vi "initialize hmac.vi"(8 "error in":errorcluster, 10 "key":string, 11 "digest name":string) -> (0 "error out":errorcluster, 3 "lvlibcrypto digest out":refnum<class "lvlibcrypto digestsign.lvclass">)   [LabVIEW 2016, in "lvlibcrypto digestsign.lvclass"]
uses:
  lvlibcrypto digestsign.lvclass
  lv tls dll.lvlib
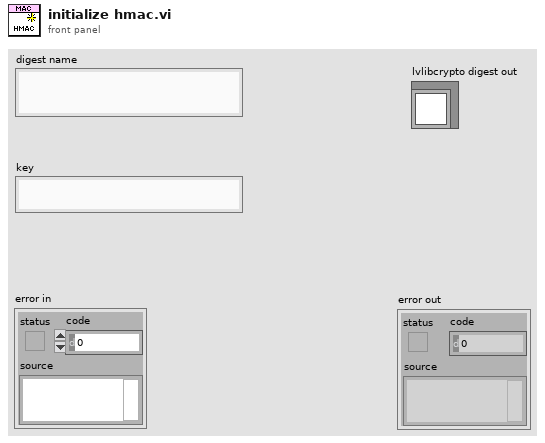
[diagram p1: front panel]
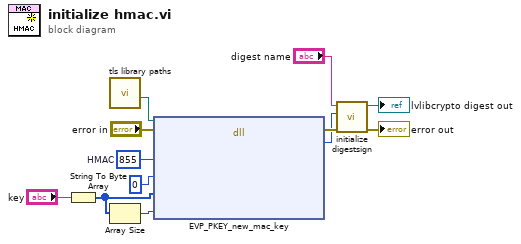
[diagram p0: block diagram]
diagram:
  w1 = 855  # HMAC
  n1 = String To Byte Array(string="key") -> (unsigned byte array=w3:u8[])
  n2 = call "tls library paths.vi"() -> ("libcrypto"=w9:path)  [unwired: 8 in, 3 out]
  n3 = Array Size(array=w3) -> (size(s)=w4:i32)
  n4 = dll-call lib="C:/Users/IEUser/Desktop/tlssimple/libcrypto-41.dll" fn="EVP_PKEY_new_mac_key"(path in=w9, error in="error in", "type"=w1, "engnull"=u64 0, "key"=w3, "keylen"=w4) -> (error out=w7:errorcluster, "pkeyptr"=w6:u64)  [unwired: 5 in, 1 out]
  n5 = call "initialize digestsign.vi"("error in"=w7, "pkey"=w6, "digest name"="digest name") -> ("error out"=→"error out":errorcluster, "lvlibcrypto digest out"=→"lvlibcrypto digest out":refnum<class "lvlibcrypto digestsign.lvclass">)  [unwired: 7 in]
